vi "cs-scanning-CLEANUP.vi"() -> ()   [LabVIEW 2017]
uses:
  raster-scan-params.ctl
  controls/PI-params.ctl
  controls/boolean_info.ctl
  controls/debug-cs.ctl
  <vilib>/rvi/Emulation/niFpgaGetClockAttributes.vi
  <vilib>/rvi/Emulation/niFpgaSctlEmulationGetInTimedLoop.vi
  <vilib>/rvi/Emulation/niFpgaEmulationReportErrorSimple.vi
  <vilib>/rvi/Emulation/niFpgaProcessEmulError.vi
  <vilib>/rvi/eio/common/nirviEmuTemplateMethod_errors.vi
  <vilib>/rvi/Emulation/niFpgaEmulationIsFPGAContextNoSignature.vi
  <vilib>/rvi/DataTransferAndStorage/Container/Common/niFpgaContainerGetUniqueNameForEmu.vi
  <vilib>/rvi/Memory/Memory_Emulation/niFpgaMemoryEmulationCacheClearOnFirstRun.vi
  <vilib>/rvi/Memory/Memory_Emulation/nirvimemoryEmulationManagerCache_MakeExclusive.vi
  <vilib>/rvi/Memory/Memory_Emulation/niFpgaMemoryEmulationValidateCache.vi
  <vilib>/rvi/Memory/Memory_Emulation/nirvimemoryEmulationManagerCache_InsertValue.vi
  <vilib>/Utility/error.llb/Clear Errors.vi
  <vilib>/rvi/Memory/Memory_Emulation/nirvimemoryEmulationManagerCache_ReleaseExclusive.vi
  <vilib>/rvi/Memory/Memory_Emulation/nirvimemoryEmulationManagerCache_GetValue.vi
  <vilib>/rvi/Memory/Memory_Emulation/nirvimemoryEmulationManagerCache_SetValue.vi
  <vilib>/rvi/DataTransferAndStorage/Container/Common/niFpgaContainerExecOnDevCompGetState.vi
  <vilib>/rvi/Emulation/niFpgaCriticalErrorInLSC.vi
  <vilib>/eio/EIONode/EIONode.xnode
  <vilib>/rvi/DataTransferAndStorage/Container/XNode/niFpgaContainer.xnode
  <vilib>/rvi/DataTransferAndStorage/Register/Emulation/niFpgaRegisterEmulation.vi
  <vilib>/rvi/DataTransferAndStorage/Register/Emulation/niFpgaRegisterEmulationRefIn.vi
  libimaging-cs.lvlib
  FPGA-data-logging.lvlib
panel:
  out "number-settled-samples-y":i16
  out "number-settled-samples-x":i16
  in  "error-threshold":sgl format="%#_13g"
  in  "settled-samples\nthreshold":i16
  in  "numEntities":i16
  in  "ABORT":bool
  in  "Ki-xy":sgl=0.001 format="%#_13g"
  in  "u_z max":sgl
  in  "xy-bound":sgl
  out "boolean indicators":T1
  out "loggin-fifo-TO":bool=TRUE
  out "input-fifo-TO":bool=TRUE
  in  "raster-scan-params":T2={"TsTicks"=1600, "Stop"=TRUE, "TOL"=0.3, "ramp-rate"=0.0, "z-u-max"=5.0, "PI-params"={"Ki"=0.001, "setpoint"=0.0}} {"z-u-max" format="%#_13g"; "TOL" format="%#_13g"}
  in  "init Z up":fxp<+/-,16,5>
  in  "u_z(0)":sgl
  out "e(0) (threshhold init)":fxp<+/-,16,5>
  in  "z_UP":fxp<+/-,16,5>
  in  "zup-N":i16
  in  "x_ffK":fxp<+/-,16,5>
  in  "trigger-0":bool
  in  "initial case":i16=2
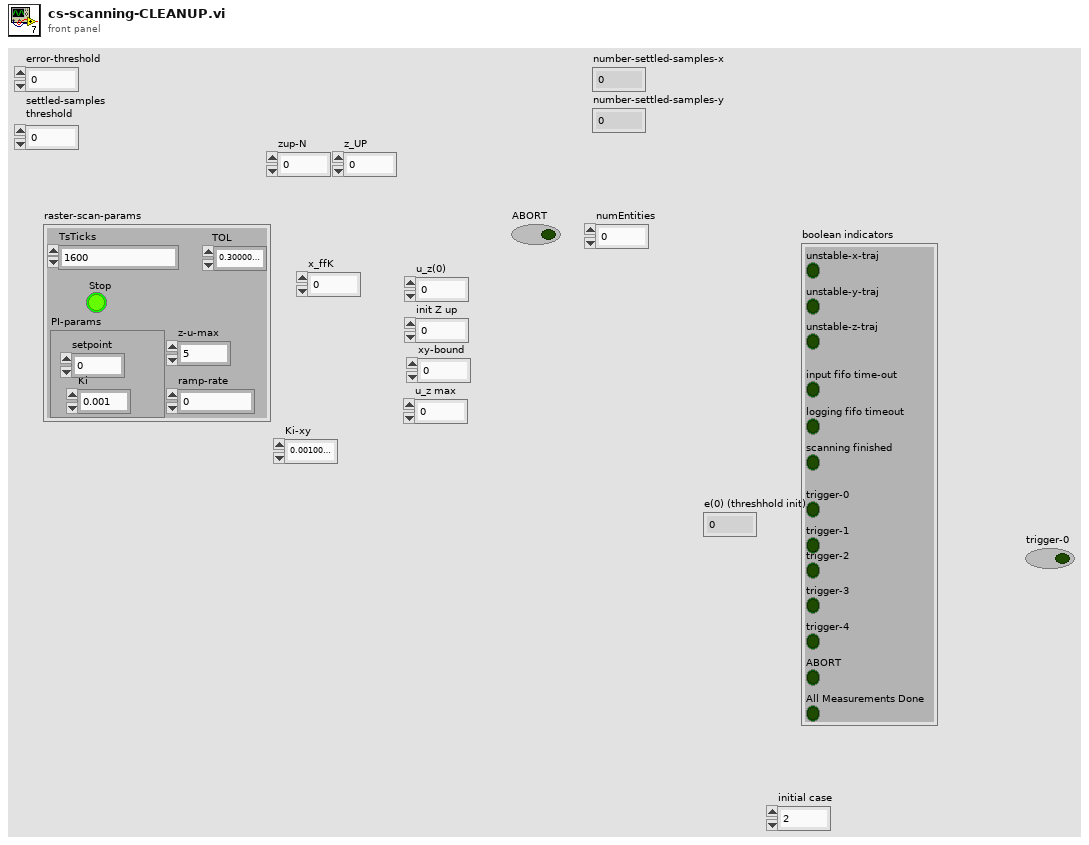
[diagram p1: front panel]
types:
  T1 = typedef "boolean_info.ctl" = cluster{"unstable-z-traj":bool, "input fifo time-out":bool, "logging fifo timeout":bool, "scanning finished":bool, "trigger-1":bool, "trigger-0":bool, "trigger-2":bool, "trigger-3":bool, "trigger-4":bool, "unstable-x-traj":bool, "unstable-y-traj":bool, "ABORT":bool, "All Measurements Done":bool}
  T2 = typedef "raster-scan-params.ctl" = cluster{"TsTicks":u32, "Stop":bool, "TOL":sgl, "ramp-rate":sgl, "z-u-max":sgl, "PI-params":T3}
  T3 = typedef "PI-params.ctl" = cluster{"Ki":sgl, "setpoint":sgl}
  T4 = typedef "debug-cs.ctl" = cluster{"ADC-zaxis":fxp<+/-,24,5>, "DAC-zaxis":sgl, "Current State":u8}
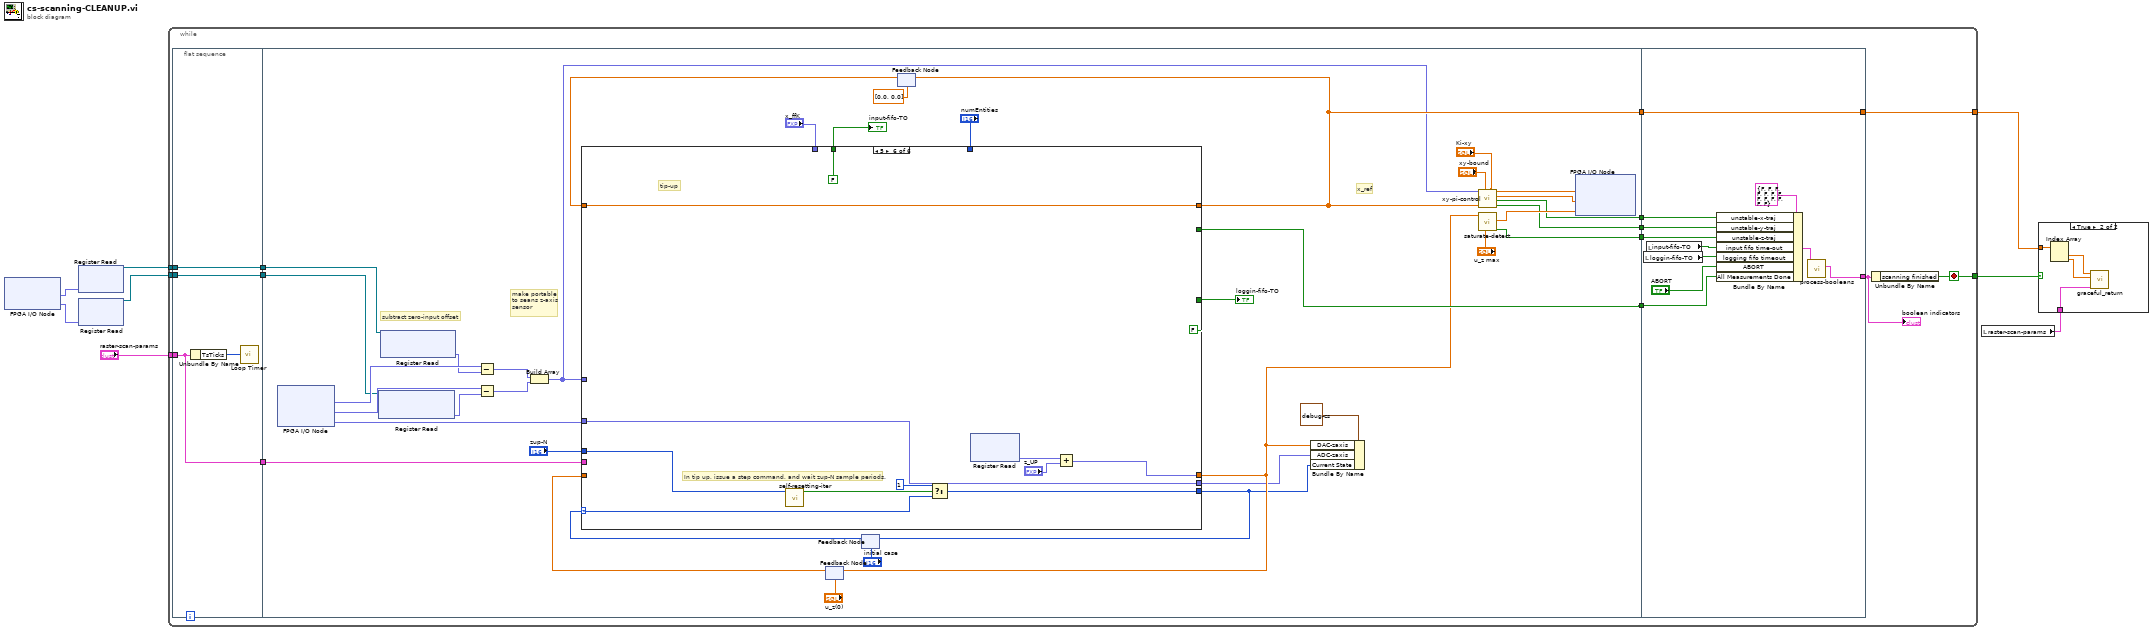
[diagram p0: block diagram]
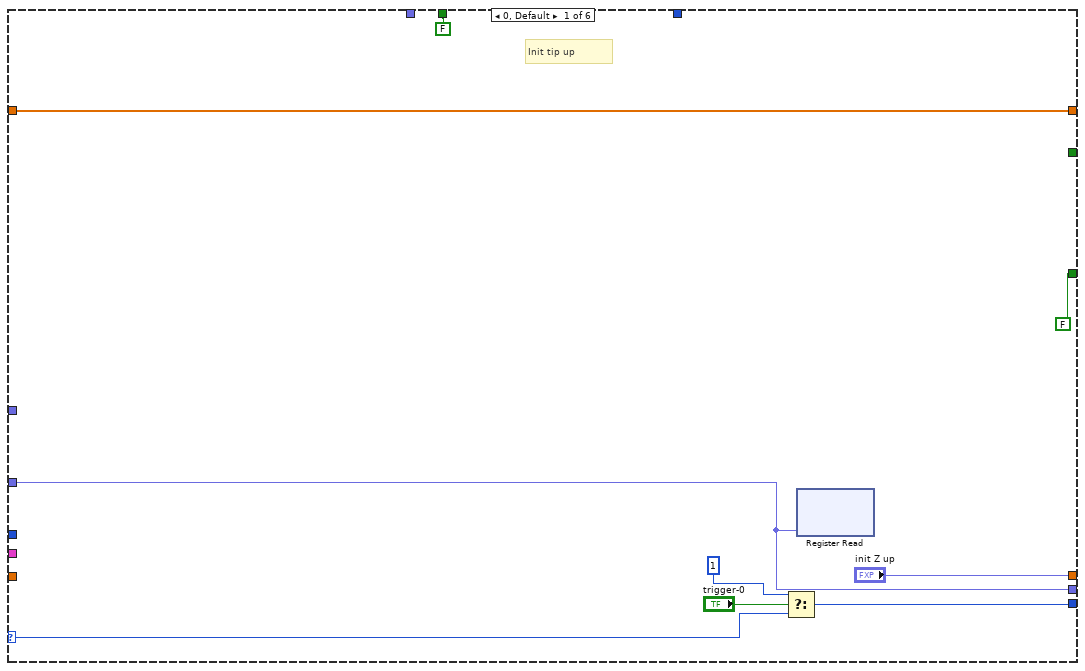
[diagram p3: hidden frame]
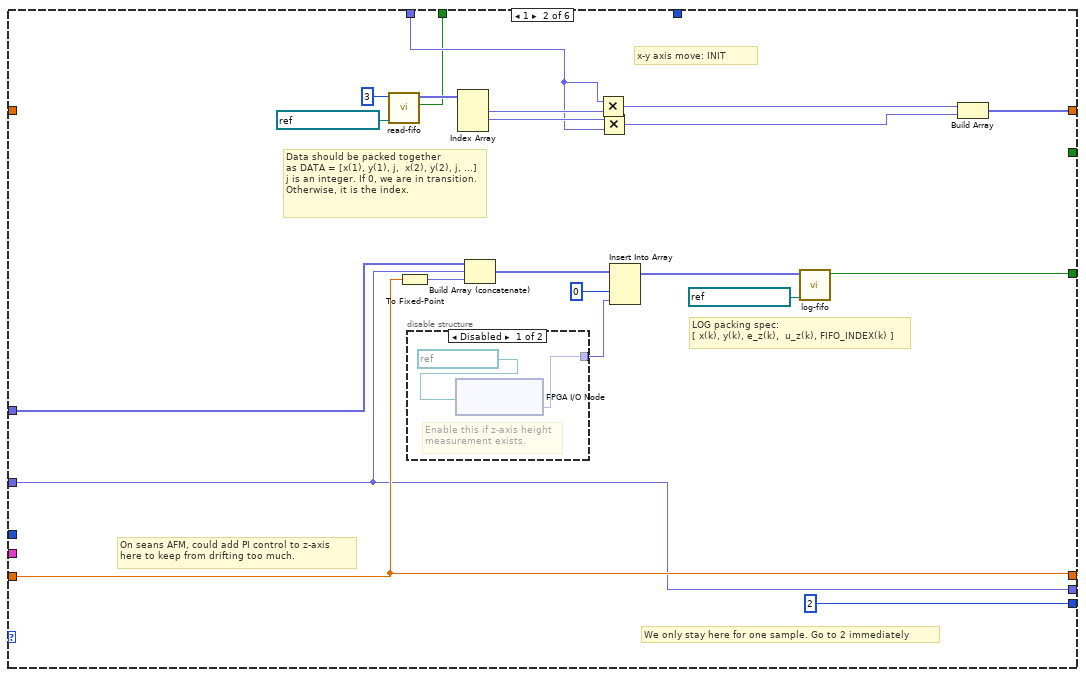
[diagram p4: hidden frame]
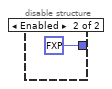
[diagram p5: hidden frame]
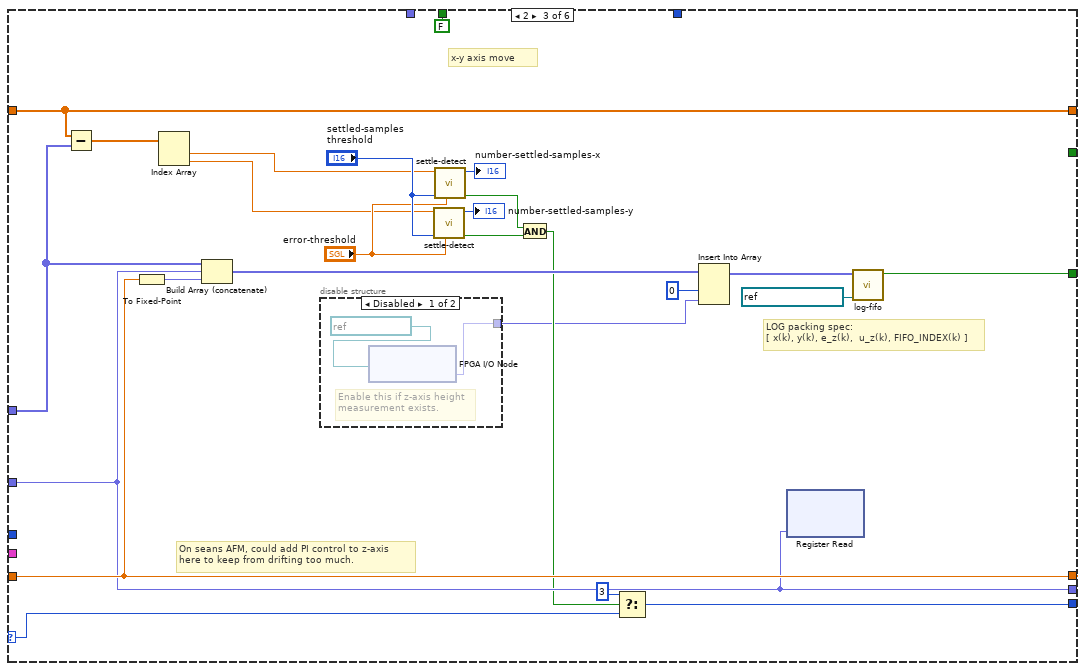
[diagram p6: hidden frame]
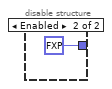
[diagram p7: hidden frame]
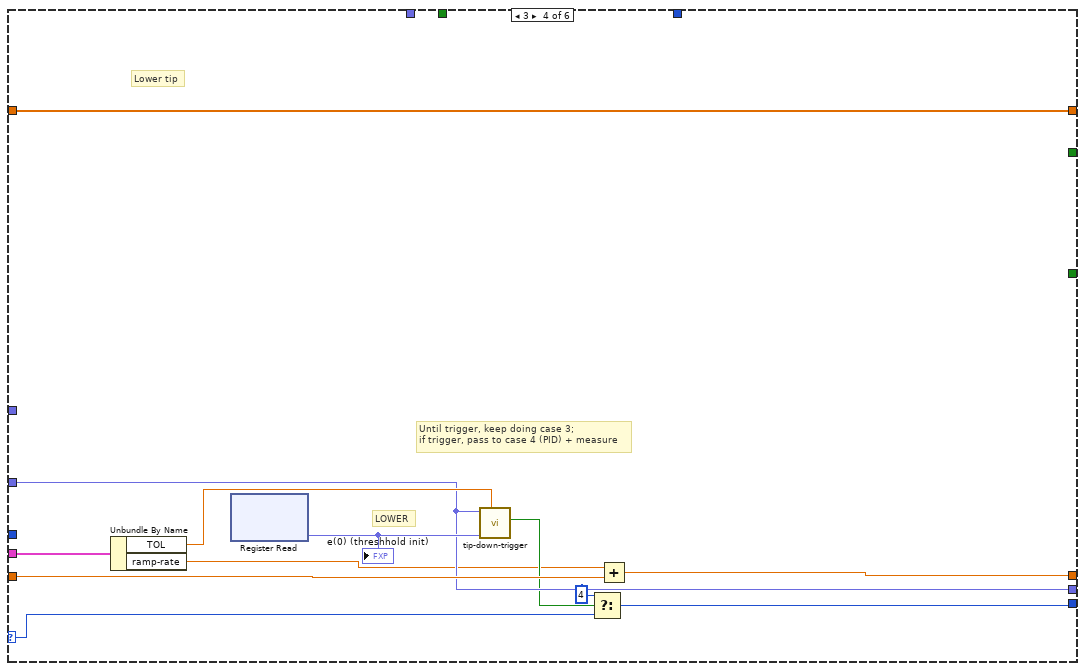
[diagram p8: hidden frame]
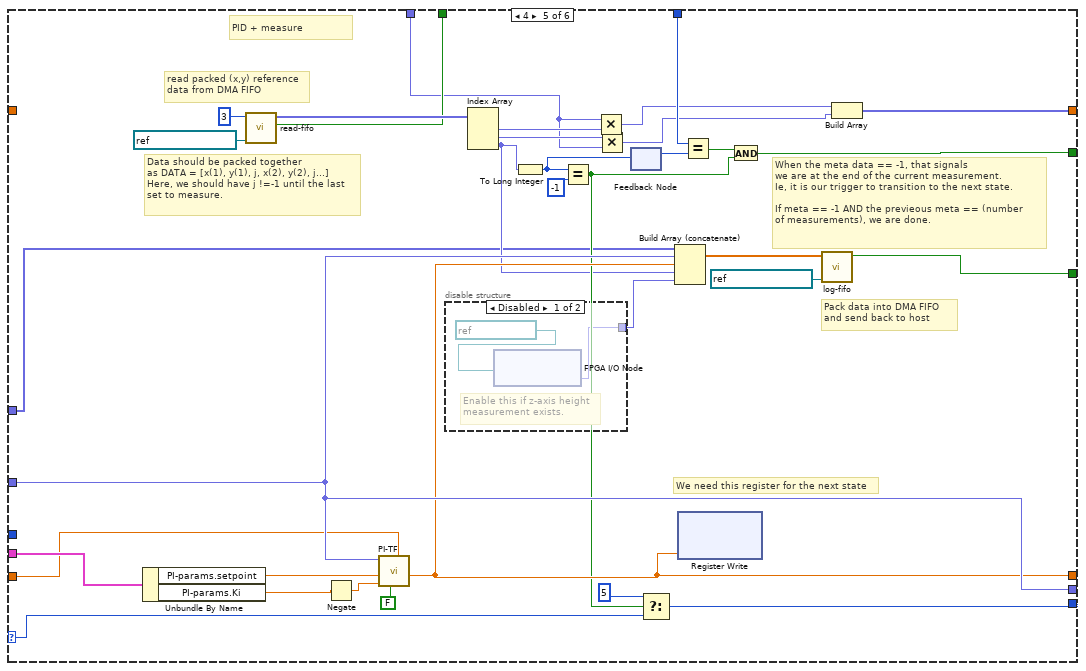
[diagram p9: hidden frame]
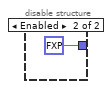
[diagram p10: hidden frame]
diagram:
  n1 = xnode "FPGA I/O Node"() -> ("Mod2/AI0"=w5:fxp<+/-,24,5>, "Mod2/AI1"=w4:fxp<+/-,24,5>)  [unwired: 2 in, 2 out]
  n2 = xnode ("Register Read")("Data"=w4) -> ("Register Out"=w2:refnum<k21>)  [unwired: 1 in]
  n3 = xnode ("Register Read")("Data"=w5) -> ("Register Out"=w3:refnum<k21>)  [unwired: 1 in]
  n4 = while {
    tunnel: "raster-scan-params" -> [w21]
    tunnel: [w20] -> w6
    tunnel: w3 -> [w14]
    tunnel: w2 -> [w12]
    tunnel: [w10] -> w1
    stop <- w20 stop-if-true
    n5 = flat-sequence {
      tunnel: w21 -> [w25]
      tunnel: [w25] -> w22
      tunnel: [w24] -> w15
      tunnel: w14 -> [w24]
      tunnel: [w23] -> w13
      tunnel: w12 -> [w23]
      tunnel: w22 -> [w56]
      tunnel: [w51] -> w18
      tunnel: [w50] -> w17
      tunnel: [w45] -> w16
      tunnel: w15 -> [w44]
      tunnel: w13 -> [w43]
      tunnel: [w31] -> w11
      tunnel: [w32] -> w9
      tunnel: [w192] -> w19
      tunnel: w18 -> [w187]
      tunnel: w17 -> [w194]
      tunnel: w16 -> [w191]
      tunnel: w11 -> [w188]
      tunnel: [w188] -> w10
      tunnel: w9 -> [w186]
      frame #0 {
        n6 = Unbundle By Name(w25) -> ("TsTicks"=w26:u32)
        n7 = call "Loop Timer"("Count(Ticks)"=w26) -> ()  [unwired: 1 out]
      }
      frame #1 {
        # "make portable\nto seans z-axis\nsensor"
        # "subtract zero-input offset"
        # "x_ref"
        n8 = xnode "FPGA I/O Node"() -> ("Mod2/AI0"=w59:fxp<+/-,24,5>, "Mod2/AI1"=w57:fxp<+/-,24,5>, "Mod2/AI2"=w61:fxp<+/-,24,5>)  [unwired: 3 in, 3 out]
        n9 = xnode ("Register Read")("Register In"=w43) -> ("Data"=w30:fxp<+/-,16,5>)  [unwired: 1 out]
        n10 = xnode ("Register Read")("Register In"=w44) -> ("Data"=w58:fxp<+/-,16,5>)  [unwired: 1 out]
        n11 = Subtract(x=w59, y=w58) -> (x-y=w29:fxp<+/-,25,6>)
        n12 = Subtract(x=w57, y=w30) -> (x-y=w28:fxp<+/-,25,6>)
        n13 = Build Array(w29, w28) -> (w27:fxp<+/-,25,6>[])
        n14 = feedback #1("u_z(0)") -> (w41:sgl)
        n15 = feedback #2("initial case") -> (w62:i16)
        n16 = feedback #3(sgl[] [0.0, 0.0]) -> (w34:sgl[])
        n17 = case shown="5" w62 {
          selector: w62 -> [w65 _ w104 w126 w153 w175]
          tunnel: [w71 i16 2 w121 w135 w169 w184] -> w37
          tunnel: w61 -> [w69 w78 w117 w130 w158 w182]
          tunnel: ["init Z up" w91 w119 w129 w151 w181] -> w39
          tunnel: w56 -> [_ _ _ w132 w163 _]
          tunnel: w41 -> [_ w91 w119 w131 w157 _]
          tunnel: [w69 w78 w117 w130 w158 w182] -> w38
          tunnel: [FALSE w81 w103 _ w141 FALSE] -> w49
          tunnel: [FALSE w84 FALSE ("timout?") _ w160 FALSE] -> w48
          tunnel: "x_ffK" -> [_ w89 _ _ w159 _]
          tunnel: "numEntities" -> [_ _ _ _ w150 _]
          tunnel: [_ _ _ _ w145 _] -> w45
          tunnel: "zup-N" -> [_ _ _ _ _ w177]
          tunnel: w34 -> [w64 _ w102 w125 _ w174]
          tunnel: [w64 w75 w102 w125 w142 w174] -> w31
          tunnel: w27 -> [_ w74 w101 _ w138 _]
          frame 0, Default {
            # "Init tip up"
            n18 = Select(t=i16 1, s="trigger-0", f=w65) -> (s? t:f=w71:i16)
            n19 = xnode ("Register Read")("Data"=w69) -> ()  [unwired: 1 in, 1 out]
          }
          frame 1 {
            # "We only stay here for one sample. Go to 2 immediately"
            # "LOG packing spec:\n[ x(k), y(k), e_z(k),  u_z(k), FIFO_INDEX(k) ]"
            # "On seans AFM, could add PI control to z-axis\nhere to keep from drifting too much."
            # "Data should be packed together\nas DATA = [x(1), y(1), j,  x(2), y(2), j, ...]\nj is an integer. If 0, we are in transition. Otherwise, it is the index."
            # "x-y axis move: INIT"
            n20 = call "read-fifo.vi"("FIFO In"=refnum<k21> "Host_to_FPGA", "numChan"=3) -> ("timout?"=w84:bool, "unpacked-data"=w85:fxp<+/-,16,5>[])  [unwired: 8 in]
            n21 = To Fixed-Point(number=w91) -> (fixed-point=w88:fxp<+/-,16,5>)  [unwired: 1 in]
            n22 = disable-structure shown="Disabled" {
              disable-tunnel: [w94 fxp<+/-,25,6> 0.0 ("new element/subarray")] -> w73
              frame Disabled {
                # "Enable this if z-axis height\nmeasurement exists."
                n23 = xnode "FPGA I/O Node"("FPGA I/O In"=refnum<k21> "Mod2/AI3") -> ("I/O Item"=w94:fxp<+/-,24,5>)  [unwired: 1 out]
              }
              frame Enabled {
              }
            }
            n24 = Index Array(array=w85) -> (element #1=w93:fxp<+/-,16,5>, element #2=w92:fxp<+/-,16,5>)  [unwired: 3 in, 1 out]
            n25 = Build Array (concatenate)(w74, w78, w88) -> (w90:fxp<+/-,25,6>[])
            n26 = Multiply(x=w89, y=w93) -> (x*y=w77:fxp<+/-,32,10>)
            n27 = Multiply(x=w92, y=w89) -> (x*y=w76:fxp<+/-,32,10>)
            n28 = Insert Into Array(array=w90, new element #1=0 ("numChan"), new element #2=w73) -> (w83:fxp<+/-,25,6>[])  [unwired: 1 in]
            n29 = call "log-fifo.vi"("FIFO In"=refnum<k21> "fpga-to-host2", "input-data"=w83) -> ("logging-timeout?"=w81:bool)  [unwired: 9 in]
            n30 = Build Array(w77, w76) -> (w75:fxp<+/-,32,10>[])
          }
          frame 2 {
            # "LOG packing spec:\n[ x(k), y(k), e_z(k),  u_z(k), FIFO_INDEX(k) ]"
            # "On seans AFM, could add PI control to z-axis\nhere to keep from drifting too much."
            # "x-y axis move"
            n31 = Subtract(x=w102, y=w101) -> (x-y=w98:sgl[])
            n32 = To Fixed-Point(number=w119) -> (fixed-point=w116:fxp<+/-,16,5>)  [unwired: 1 in]
            n33 = Index Array(array=w98) -> (element #1=w99:sgl, element #2=w100:sgl)  [unwired: 2 in]
            n34 = Build Array (concatenate)(w101, w117, w116) -> (w118:fxp<+/-,25,6>[])
            n35 = disable-structure shown="Disabled" {
              disable-tunnel: [w122 fxp<+/-,25,6> 0.0 ("new element/subarray")] -> w97
              frame Disabled {
                # "Enable this if z-axis height\nmeasurement exists."
                n36 = xnode "FPGA I/O Node"("FPGA I/O In"=refnum<k21> "Mod2/AI3") -> ("I/O Item"=w122:fxp<+/-,24,5>)  [unwired: 1 out]
              }
              frame Enabled {
              }
            }
            n37 = call "settle-detect.vi"("error-max"="error-threshold", "settled-samples\nthreshold"="settled-samples\nthreshold", "err(k)"=w100) -> ("has-settled"=w111:bool, "number-settled-samples"=→"number-settled-samples-y":i16)  [unwired: 7 in]
            n38 = call "settle-detect.vi"("error-max"="error-threshold", "settled-samples\nthreshold"="settled-samples\nthreshold", "err(k)"=w99) -> ("has-settled"=w110:bool, "number-settled-samples"=→"number-settled-samples-x":i16)  [unwired: 7 in]
            n39 = And(x=w110, y=w111) -> (x .and. y?=w107:bool)
            n40 = Select(t=i16 3, s=w107, f=w104) -> (s? t:f=w121:i16)
            n41 = Insert Into Array(array=w118, new element #1=i16 0, new element #2=w97) -> (w115:fxp<+/-,25,6>[])  [unwired: 1 in]
            n42 = xnode ("Register Read")("Data"=w117) -> ()  [unwired: 1 in, 1 out]
            n43 = call "log-fifo.vi"("FIFO In"=refnum<k21> "fpga-to-host2", "input-data"=w115) -> ("logging-timeout?"=w103:bool)  [unwired: 9 in]
          }
          frame 3 {
            # "Until trigger, keep doing case 3;\nif trigger, pass to case 4 (PID) + measure"
            # "LOWER"
            # "Lower tip"
            n44 = Unbundle By Name(w132) -> ("TOL"=w133:sgl, "ramp-rate"=w127:sgl)
            n45 = xnode ("Register Read")() -> ("Data"=w134:fxp<+/-,16,5>)  [unwired: 1 in, 1 out]
            "e(0) (threshhold init)" <- w134
            n46 = call "tip-down-trigger.vi"("TOL"=w133, "Vo"=w134, "e(k)"=w130) -> ("trigger"=w128:bool)  [unwired: 8 in]
            n47 = Select(t=i16 4, s=w128, f=w126) -> (s? t:f=w135:i16)
            n48 = Add(x=w127, y=w131) -> (x+y=w129:sgl)
          }
          frame 4 {
            # "Pack data into DMA FIFO\nand send back to host"
            # "read packed (x,y) reference\ndata from DMA FIFO"
            # "When the meta data == -1, that signals\nwe are at the end of the current measurement.\nIe, it is our trigger to transition to the next state.\n\nIf meta == -1 AND the previeous meta == (number\nof measurements), we are done."
            # "We need this register for the next state"
            # "Data should be packed together\nas DATA = [x(1), y(1), j, x(2), y(2), j...]\nHere, we should have j !=-1 until the last\nset to measure."
            # "PID + measure"
            n49 = Unbundle By Name(w163) -> ("PI-params.setpoint"=w164:sgl, "PI-params.Ki"=w161:sgl)
            n50 = call "read-fifo.vi"("FIFO In"=refnum<k21> "Host_to_FPGA", "numChan"=3) -> ("timout?"=w160:bool, "unpacked-data"=w166:fxp<+/-,16,5>[])  [unwired: 8 in]
            n51 = Negate(x=w161) -> (-x=w162:sgl)
            n52 = call "PI-TF.vi"("u(k-1)"=w157, "reset"=FALSE, "Ki"=w162, "setpoint"=w164, "y(k)"=w158) -> ("u(k)"=w151:sgl)  [unwired: 6 in]
            n53 = disable-structure shown="Disabled" {
              disable-tunnel: [w171 fxp<+/-,25,6> 0.0 ("new element/subarray")] -> w137
              frame Disabled {
                # "Enable this if z-axis height\nmeasurement exists."
                n54 = xnode "FPGA I/O Node"("FPGA I/O In"=refnum<k21> "Mod2/AI3") -> ("I/O Item"=w171:fxp<+/-,24,5>)  [unwired: 1 out]
              }
              frame Enabled {
              }
            }
            n55 = Index Array(array=w166) -> (element #1=w168:fxp<+/-,16,5>, element #2=w167:fxp<+/-,16,5>, element #3=w140:fxp<+/-,16,5>)  [unwired: 3 in]
            n56 = To Long Integer(number=w140) -> (32bit integer=w148:i32)
            n57 = Equal?(x=w148, y=-1) -> (x = y?=w146:bool)
            n58 = Multiply(x=w159, y=w168) -> (x*y=w144:fxp<+/-,32,10>)
            n59 = Multiply(x=w167, y=w159) -> (x*y=w143:fxp<+/-,32,10>)
            n60 = feedback-in #4(w148) -> ()
            n61 = feedback #4() -> (w149:i32)  [unwired: 1 in]
            n62 = Select(t=i16 5, s=w146, f=w153) -> (s? t:f=w169:i16)
            n63 = Build Array (concatenate)(w138, w158, w151, w140, w137) -> (w139:sgl[])
            n64 = xnode ("Register Write")("Data"=w151) -> ()  [unwired: 1 in, 1 out]
            n65 = Equal?(x=w150, y=w149) -> (x = y?=w147:bool)
            n66 = And(x=w147, y=w146) -> (x .and. y?=w145:bool)
            n67 = call "log-fifo.vi"("FIFO In"=refnum<k21> "fpga-to-host2", "input-data"=w139) -> ("logging-timeout?"=w141:bool)  [unwired: 9 in]
            n68 = Build Array(w144, w143) -> (w142:fxp<+/-,32,10>[])
          }
          frame 5 {
            # "In tip up, issue a step command, and wait zup-N sample periods."
            # "tip-up"
            n69 = call "self-resetting-iter.vi"("N"=w177) -> ("Boolean"=w176:bool)  [unwired: 9 in, 1 out]
            n70 = Select(t=i16 1, s=w176, f=w175) -> (s? t:f=w184:i16)
            n71 = xnode ("Register Read")() -> ("Data"=w179:fxp<+/-,16,5>)  [unwired: 1 in, 1 out]
            n72 = Add(x=w179, y="z_UP") -> (x+y=w181:fxp<+/-,17,6>)
          }
        }
        "loggin-fifo-TO" <- w49
        "input-fifo-TO" <- w48
        n73 = feedback-in #1(w39) -> ()
        n74 = feedback-in #2(w37) -> ()
        n75 = feedback-in #3(w31) -> ()
        n76 = Bundle By Name(cluster=T4 {"ADC-zaxis"=0.0, "DAC-zaxis"=0.0, "Current State"=0} ("debug"), "DAC-zaxis"=w39, "ADC-zaxis"=w38, "Current State"=w37) -> ()  [unwired: 1 out]
        n77 = call "xy-pi-control.vi"("Ki-xy"="Ki-xy", "xy-umax"="xy-bound", "xy-ref"=w31, "x_k-y_k"=w27) -> ("u_y saturated"=w32:bool, "u_x saturated"=w51:bool, "sat(u_y)"=w55:sgl, "sat(u_x)"=w54:sgl)  [unwired: 4 in]
        n78 = call "saturate-detect.vi"("bound"="u_z max", "x"=w39) -> ("saturated"=w50:bool, "sat(x)"=w53:sgl)  [unwired: 8 in]
        n79 = xnode "FPGA I/O Node"("Mod1/AO0"=w54, "Mod1/AO1"=w55, "Mod1/AO2"=w53) -> ()  [unwired: 3 in, 3 out]
      }
      frame #2 {
        n80 = local read "loggin-fifo-TO"() -> (w195:bool)
        n81 = local read "input-fifo-TO"() -> (w196:bool)
        n82 = Bundle By Name(cluster=T1 {"unstable-z-traj"=FALSE, "input fifo time-out"=FALSE, "logging fifo timeout"=FALSE, "scanning finished"=FALSE, "trigger-1"=FALSE, "trigger-0"=FALSE, "trigger-2"=FALSE, "trigger-3"=FALSE, "trigger-4"=FALSE, "unstable-x-traj"=FALSE, "unstable-y-traj"=FALSE, "ABORT"=FALSE, "All Measurements Done"=FALSE} ("boolean errors"), "unstable-x-traj"=w187, "unstable-y-traj"=w186, "unstable-z-traj"=w194, "input fifo time-out"=w196, "logging fifo timeout"=w195, "ABORT"="ABORT", "All Measurements Done"=w191) -> (w190:T1)
        n83 = call "process-booleans.vi"("boolean indicators 2"=w190) -> ("boolean indicators"=w192:T1)  [unwired: 10 in]
      }
    }
    n84 = Unbundle By Name(w19) -> ("scanning finished"=w20:bool)
    "boolean indicators" <- w19
  }
  n85 = local read "raster-scan-params"() -> (w7:T2)
  n86 = case shown="True" w6 {
    tunnel: w7 -> [_ w200]
    tunnel: w1 -> [_ w199]
    frame False {
    }
    frame True {
      n87 = Index Array(array=w199) -> (element #1=w198:sgl, element #2=w197:sgl)  [unwired: 2 in]
      n88 = call "graceful_return.vi"("raster-scan-params"=w200, "uy(0)"=w197, "ux(0)"=w198) -> ()  [unwired: 9 in]
    }
  }
